vi "Blob Detection.vi"() -> ()   [LabVIEW 2018]
uses:
  <vilib>/Platform/TimedLoop/XDataNode/timing_clust.ctl
  <vilib>/Platform/TimedLoop/XDataNode/nitl_modes.ctl
  <vilib>/Platform/TimedLoop/XDataNode/wakeup.ctl
  <vilib>/Platform/TimedLoop/XDataNode/XDataNode.xnode
  <vilib>/vision/NI_Vision_Development_Module.lvlib
  <vilib>/Platform/TimedLoop/XDataNode/XDNodeRunTimeDep.lvlib
panel:
  in  "Threshold Range":sgl(slide)=20.041805 scale=0.0..255.0
  out "Error Out":errorcluster
  out "Original Image":T1(plugin-control)
  in  "Stop Button":bool
  in  "Connectivity":enum16{"8", "4"}(ring)
  in  "Image Source":enum16{"Static ", "Camera"}(ring)
  out "Calibrated":bool
  out "Processed Image":T1(plugin-control)
  out "Grayscale Intensity Histogram":u32[](graph)
  out "Number of Particles":i32
  out "Particle Reports (Pixels)":T2(array[cluster])
  # "Mechatronic Systems Board"
  # "Blob Detection"
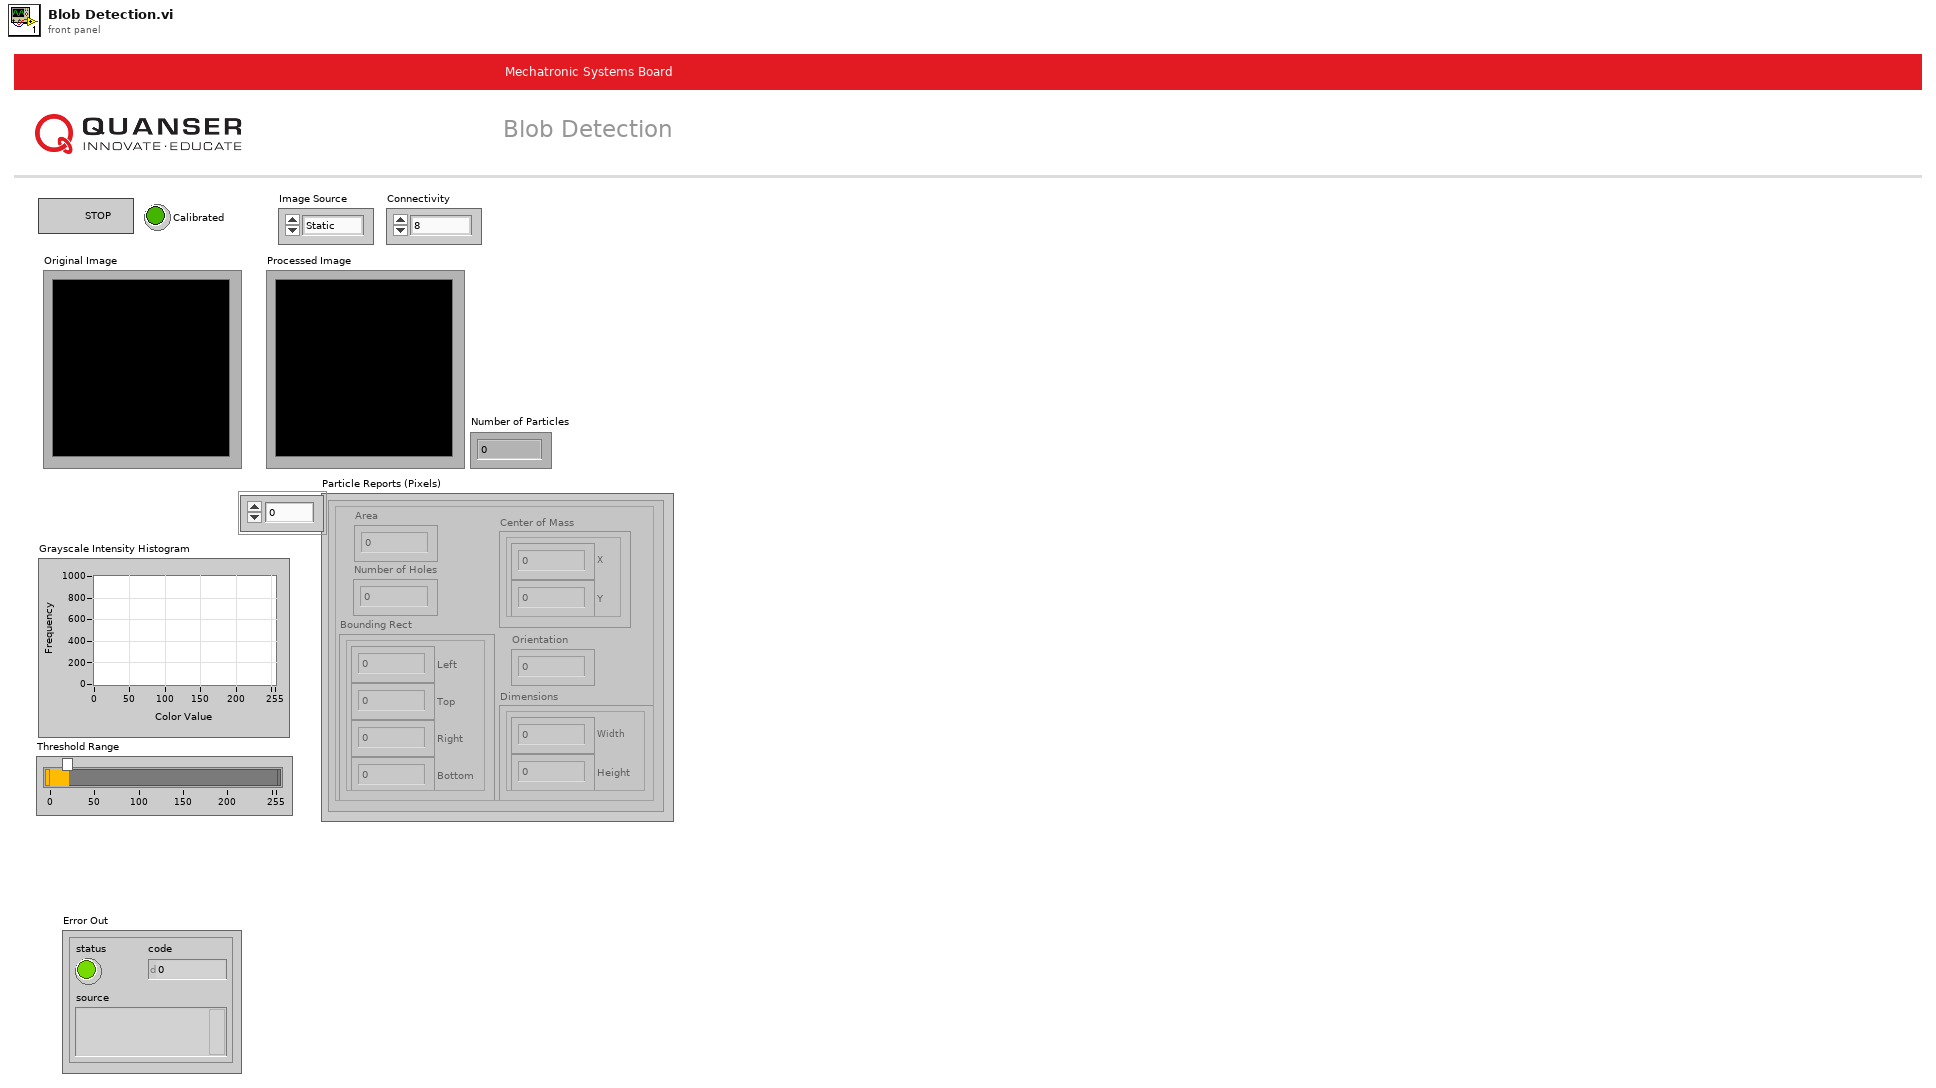
[diagram p1: front panel]
types:
  T1 = typedef "IMAQ Image.ctl" = refnum<image>
  T2 = cluster{"Area":dbl, "Number of Holes":dbl, "Bounding Rect":cluster{"Left":dbl, "Top":dbl, "Right":dbl, "Bottom":dbl}, "Center of Mass":cluster{"X":dbl, "Y":dbl}, "Orientation":dbl, "Dimensions":cluster{"Width":dbl, "Height":dbl}}[]
  T3 = typedef "QNET MS IO Cluster.ctl" = cluster{"Error":errorcluster, "Encoder Calibration Values":i32[], "Update Calibration":bool, "JPEG Resolutions":u16, "Raw Resolutions":u16, "Image Mode":enum16{"RAW RGB", "RAW Gray Scale", "JPEG"}, "FPGA Ref":refnum<k20>}
  T4 = typedef "XDNodeRunTimeDep.lvlib/timing_clust.ctl" = cluster{"Expected End [f-1]":u64, "Actual End [f-1]":u64, "Finished Late? [f-1]":bool, "Expected End [i-1]":u64, "Actual End [i-1]":u64, "Finished Late? [i-1]":bool, "Expected Start [i]":u64, "Actual Start [i]":u64, "Expected Start [f]":u64, "Actual Start [f]":u64, "Source Name":string, "Structure Name":string, "Period":i64, "Deadline":i64, "Offset":i64, "Start":i64, "Priority":i32, "Timeout":i32, "Mode":T5, "Wakeup Reason":T6, "Error":errorcluster, "Source Type":string, "Secondary Source Type":string, "Global End Time":u64, "Global Start Time":u64, "Frame Duration":u64, "Iteration Duration":u64, "Assigned CPU":i32, "I/O Scan Engine Mode":u32}
  T5 = typedef "XDNodeRunTimeDep.lvlib/nitl_modes.ctl" = enum32{"No Change", "Process missed periods, maintain original phase", "Discard missed periods, maintain original phase", "Process missed periods, ignore original phase", "Discard missed periods, ignore original phase"}
  T6 = typedef "XDNodeRunTimeDep.lvlib/wakeup.ctl" = enum32{"Normal", "Aborted", "Asynchronous wakeup", "Timing source error", "Timed loop error", "Timeout"}
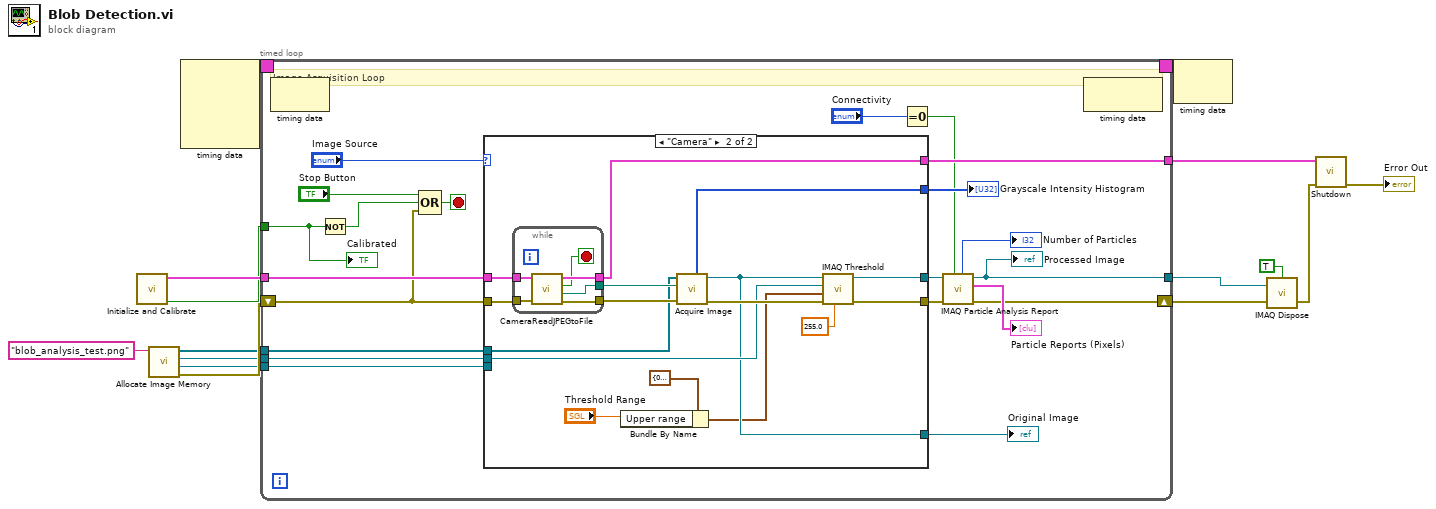
[diagram p0: block diagram]
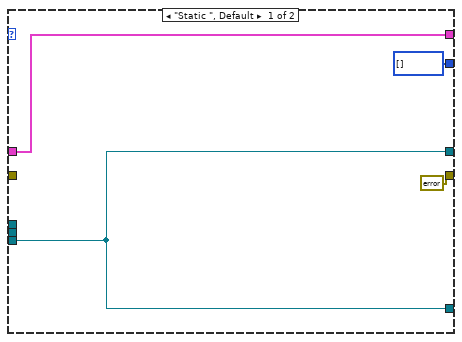
[diagram p2: hidden frame]
diagram:
  n1 = call "Initialize and Calibrate.vi"() -> ("Calibrated"=w11:bool, "IO Cluster"=w12:T3)  [unwired: 10 in]
  n2 = call "Allocate Image Memory.vi"("Reference Image File"="blob_analysis_test.png") -> ("error out"=w5:errorcluster, "Reference Image"=w2:T1, "HSL Threshold"=w3:T1, "Acquisition Memory"=w1:T1[])  [unwired: 5 in, 2 out]
  n3 = node-c288() -> (w9:T4)  [unwired: 4 in]
  n4 = timed-loop {
    tunnel: [w34] -> w14
    tunnel: [w29] -> w13
    tunnel: w12 -> [w23]
    tunnel: w11 -> [w36]
    timing: w9 -> [_]
    timing-out: [_] -> w8
    tunnel: w3 -> [w22]
    shift-right: [w27] -> w7
    shift-left: w5 -> [w19]
    tunnel: w2 -> [w17]
    tunnel: w1 -> [w16]
    stop <- w18 stop-if-true
    # "Image Acquisition Loop"
    n5 = node-c288() -> ()  [unwired: 1 in, 1 out]
    n6 = Not(x=w36) -> (.not. x?=w20:bool)
    n7 = Compound Arithmetic op=OR("Stop Button", w20, w19) -> (w18:bool)
    n8 = case shown="\"Camera\"" "Image Source" {
      tunnel: [w39 w56] -> w31
      tunnel: [errorcluster {"status"=FALSE, "code"=0, "source"=""} ("Error Out") w55] -> w30
      tunnel: w23 -> [w41 w53]
      tunnel: w17 -> [w39 _]
      tunnel: [u32[] [] ("histogram") w58] -> w35
      tunnel: [w39 w49] -> w24
      tunnel: [w41 w52] -> w34
      tunnel: w22 -> [_ w50]
      tunnel: w19 -> [_ w48]
      tunnel: w16 -> [_ w46]
      frame "Static ", Default {
      }
      frame "Camera" {
        n9 = while {
          tunnel: [w60] -> w47
          tunnel: w53 -> [w64]
          tunnel: [w63] -> w52
          tunnel: w48 -> [w61]
          tunnel: [w62] -> w51
          stop <- w59 stop-if-true
          n10 = call "CameraReadJPEGtoFile.vi"("error in"=w61, "IO Cluster In"=w64) -> ("Error Out"=w62:errorcluster, "Image File"=w60:path, "New Image Data"=w59:bool, "IO Cluster Out"=w63:T3)  [unwired: 6 in]
        }
        n11 = Bundle By Name(cluster=cluster{"Lower range":sgl, "Upper range":sgl} {"Lower range"=0.0, "Upper range"=255.0} ("input cluster"), "Upper range"="Threshold Range") -> (w44:cluster{"Lower range":sgl, "Upper range":sgl})
        n12 = call "Acquire Image.vi"("Error In"=w51, "File Path"=w47, "Acquisition Memory"=w46) -> ("Error Out"=w57:errorcluster, "Pre-processed Image"=w49:T1, "histogram"=w58:u32[])  [unwired: 4 in, 2 out]
        n13 = call "IMAQ Threshold"("Replace Value"=sgl 255.0, "error in (no error)"=w57, "Range"=w44, "Image Dst"=w50, "Image Src"=w49) -> ("error out"=w55:errorcluster, "Image Dst Out"=w56:T1)  [unwired: 5 in]
      }
    }
    "Grayscale Intensity Histogram" <- w35
    "Original Image" <- w24
    n14 = Equal To 0?(x="Connectivity") -> (x = 0?=w26:bool)
    n15 = call "IMAQ Particle Analysis Report"("Connectivity 4/8 (8)"=w26, "error in (no error)"=w30, "Image"=w31) -> ("error out"=w27:errorcluster, "Particle Reports (Pixels)"=→"Particle Reports (Pixels)":T2, "Image Out (duplicate)"=w29:T1, "Number of Particles"=→"Number of Particles":i32)  [unwired: 3 in, 2 out]
    "Processed Image" <- w29
    n16 = node-c288() -> ()  [unwired: 1 in, 1 out]
    "Calibrated" <- w36
  }
  n17 = node-c288(w8) -> ()  [unwired: 1 out]
  n18 = call "IMAQ Dispose"("All Images? (No)"=TRUE, "Image"=w13, "error in (no error)"=w7) -> ("error out"=w15:errorcluster)  [unwired: 3 in]
  n19 = call "Shutdown.vi"("Image Processing Loop"=w15, "IO Cluster In"=w14) -> ("Error"=→"Error Out":errorcluster)  [unwired: 9 in]
